vi "Send Message.vi"(7 "Priority Message":bool, 8 "error in":errorcluster, 9 "Payload":variant, 10 "Command":string) -> (0 "error out":errorcluster)   [LabVIEW 2020, in "Hardware.lvlib"]
uses:
  Hardware.lvlib
  Messaging/Message Type.ctl
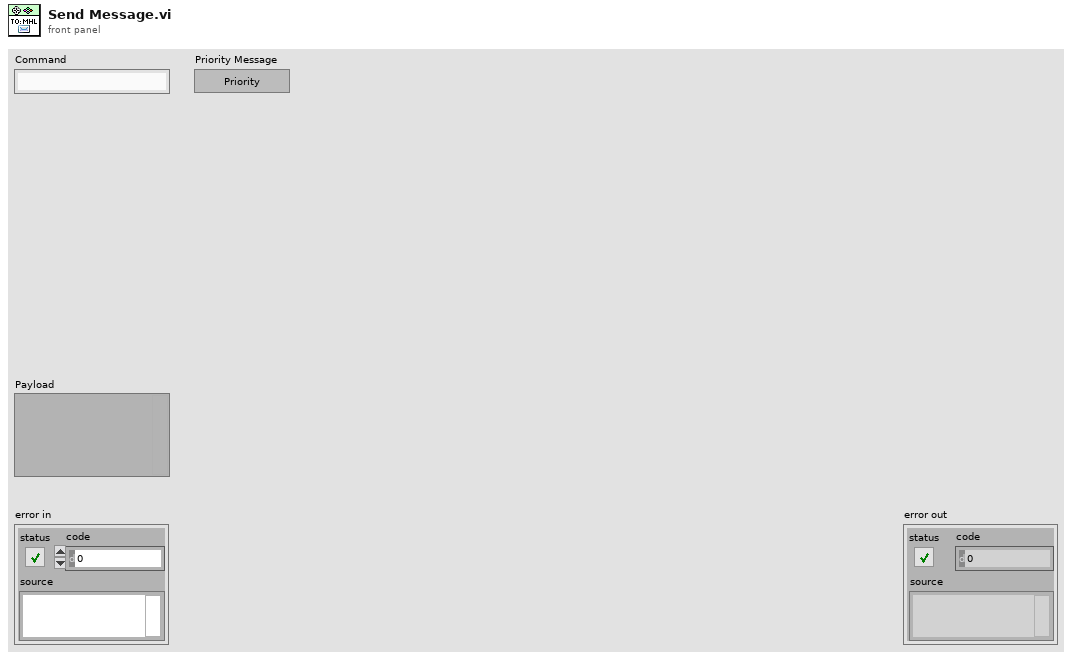
[diagram p1: front panel]
types:
  T1 = typedef "Hardware.lvlib/Message Type.ctl" = cluster{"Command":string, "Payload":variant}
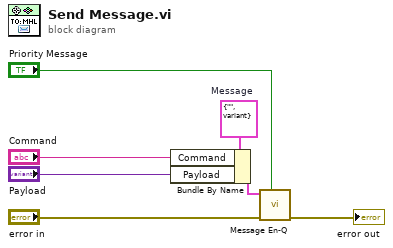
[diagram p0: block diagram]
diagram:
  w2 = T1 {"Command"="", "Payload"=variant}  # Message
  n1 = Bundle By Name(cluster=w2, "Command"="Command", "Payload"="Payload") -> (w5:T1)
  n2 = call "Message En-Q.vi"("Priority Message"="Priority Message", "error in"="error in", "Message Q Type"=w5) -> ("error out"=→"error out":errorcluster)  [unwired: 8 in]
